vi "String Message add.vi"(4 "Datetime Format":enum16{"Full", "HH:MM:SS"}(ring), 5 "Display":bool=TRUE, 6 "Clear":bool, 7 "String Length":i32=2000, 8 "error in (no error)":errorcluster, 9 "String":string, 10 "Main":string, 11 "Messages":refnum<vi>) -> (0 "error out":errorcluster, 2 "String 2":string, 3 "reference out":refnum<vi>)   [LabVIEW 2021]
doc: "为顶层UI的Message里面累计添加信息。最新的在最上面"
uses:
  <userlib>/sushu/sushu.lvlib
  Z:/UTP_2023/Source_Public/DataBase/DataBase_SQL/DataBase_SQL.lvclass
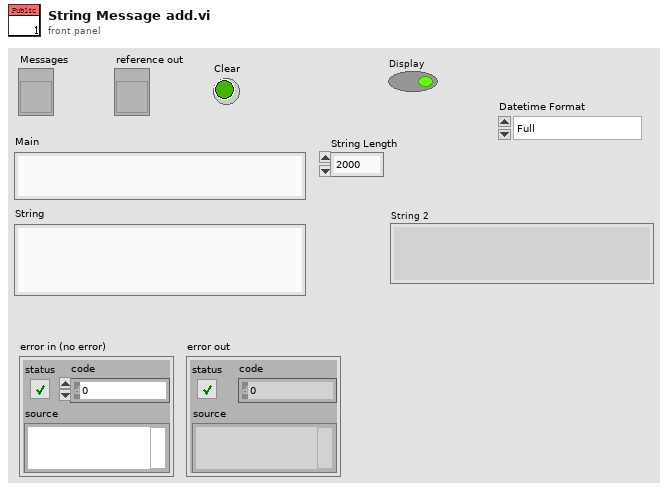
[diagram p1: front panel]
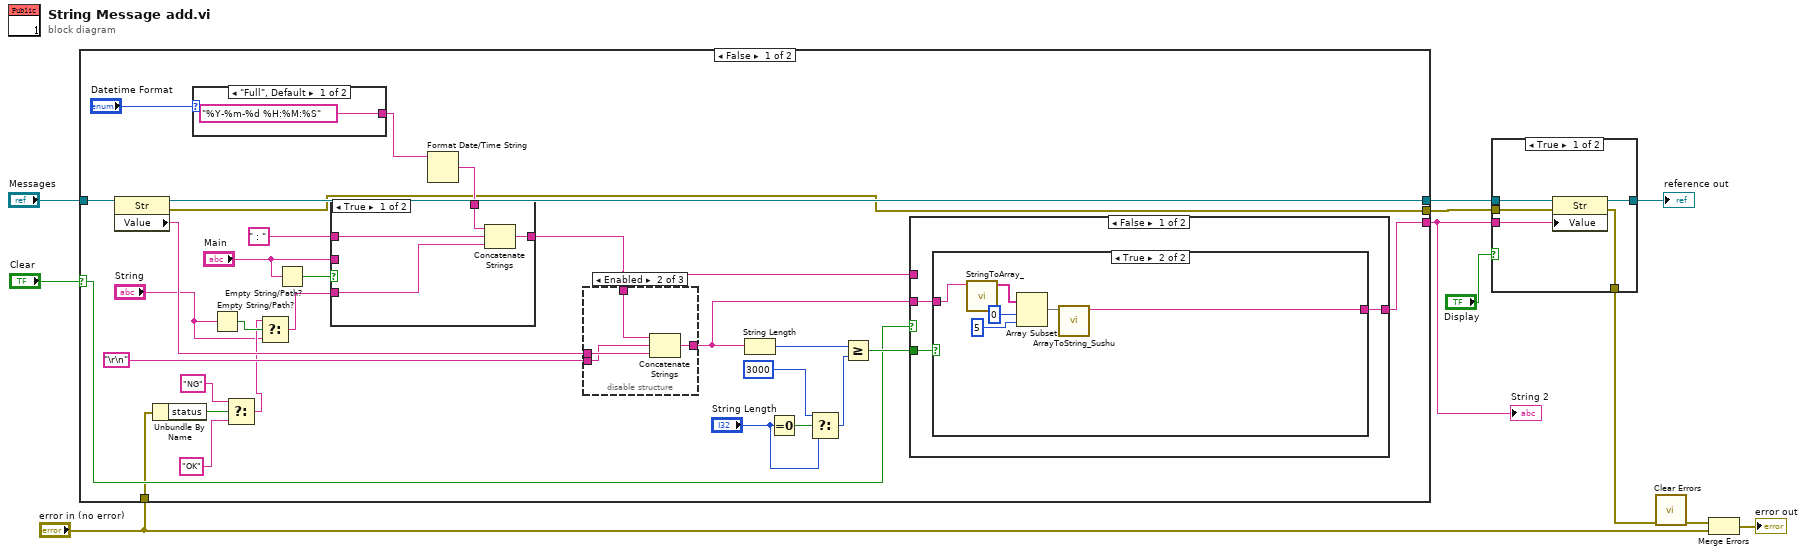
[diagram p0: block diagram]
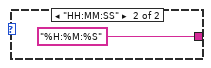
[diagram p3: hidden frame]
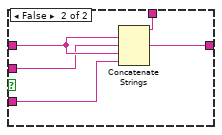
[diagram p6: hidden frame]
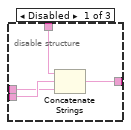
[diagram p7: hidden frame]
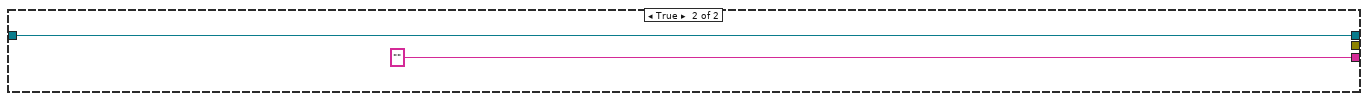
[diagram p9: hidden frame]
diagram:
  n1 = case shown="False" "Clear" {
    selector: "Clear" -> [w24 _]
    tunnel: "Messages" -> [w40 w72]
    tunnel: [w37 w72] -> w10
    tunnel: [w29 "" ("String")] -> w8
    tunnel: "error in (no error)" -> [w22 _]
    tunnel: [w14 _] -> w5
    frame False {
      n2 = property class="Str"(reference=w40) -> (reference out=w37:refnum<vi>, error out=w14:errorcluster, "Value"=w38:string)  [unwired: 1 in]
      n3 = Unbundle By Name(w22) -> ("status"=w21:bool)
      n4 = case shown="\"Full\", Default" "Datetime Format" {
        tunnel: ["%Y-%m-%d %H:%M:%S" ("time format string (%c)") "%H:%M:%S" ("time format string (%c)")] -> w12
        frame "Full", Default {
        }
        frame "HH:MM:SS" {
        }
      }
      n5 = Empty String/Path?(string/path="String") -> (empty?=w18:bool)
      n6 = Select(t="NG" ("string"), s=w21, f="OK" ("string")) -> (s? t:f=w17:string)
      n7 = Select(t=w17, s=w18, f="String") -> (s? t:f=w15:string)
      n8 = Empty String/Path?(string/path="Main") -> (empty?=w26:bool)
      n9 = Format Date/Time String(time format string (%c)=w12) -> (date/time string=w36:string)  [unwired: 2 in]
      n10 = case shown="True" w26 {
        tunnel: [w57 w62] -> w23
        tunnel: w36 -> [w56 w61]
        tunnel: " : " ("string") -> [w55 w60]
        tunnel: w15 -> [w54 w59]
        tunnel: "Main" -> [_ w58]
        frame True {
          n11 = Concatenate Strings(w56, w55, w54) -> (w57:string)
        }
        frame False {
          n12 = Concatenate Strings(w61, w60, w58, w60, w59) -> (w62:string)
        }
      }
      n13 = disable-structure shown="Enabled" {
        disable-tunnel: "\r\n" -> [w66 w68 _]
        disable-tunnel: w38 -> [w65 w70 _]
        disable-tunnel: [w64 w69 _] -> w30
        disable-tunnel: w23 -> [w63 w67 _]
        frame Disabled {
          n14 = Concatenate Strings(w63, w66, w65) -> (w64:string)
        }
        frame Enabled {
          n15 = Concatenate Strings(w67, w68, w70) -> (w69:string)
        }
        frame Disabled {
        }
      }
      n16 = String Length(string=w30) -> (length=w35:i32)
      n17 = Equal To 0?(x="String Length") -> (x = 0?=w34:bool)
      n18 = Select(t=3000 ("y"), s=w34, f="String Length") -> (s? t:f=w31:i32)
      n19 = Greater Or Equal?(x=w35, y=w31) -> (x >= y?=w25:bool)
      n20 = case shown="False" w24 {
        tunnel: w30 -> [w45 _]
        tunnel: [w44 w53] -> w29
        tunnel: w25 -> [w43 _]
        tunnel: w23 -> [_ w53]
        frame False {
          n21 = case shown="True" w43 {
            tunnel: w45 -> [w46 w48]
            tunnel: [w46 w49] -> w44
            frame False {
            }
            frame True {
              n22 = call "StringToArray_.vi"("State Queue"=w48) -> ("Array"=w47:string[])  [unwired: 7 in, 3 out]
              n23 = Array Subset(array=w47, index=0, length=5) -> (w50:string[])
              n24 = call <userlib>:"ArrayToString_Sushu.vi"("Array"=w50) -> ("String"=w49:string)  [unwired: 10 in]
            }
          }
        }
        frame True {
        }
      }
    }
    frame True {
    }
  }
  "String 2" <- w8
  n25 = case shown="True" "Display" {
    tunnel: w10 -> [w77 w79]
    tunnel: [w76 w79] -> w9
    tunnel: w8 -> [w75 _]
    tunnel: w5 -> [w74 w78]
    tunnel: [w73 w78] -> w3
    frame True {
      n26 = property class="Str"(reference=w77, error in=w74, "Value"=w75) -> (reference out=w76:refnum<vi>, error out=w73:errorcluster)
    }
    frame False {
    }
  }
  "reference out" <- w9
  n27 = call <vilib>:"Clear Errors.vi"("error in (no error)"=w3) -> ("error out"=w2:errorcluster)  [unwired: 5 in, 1 out]
  n28 = Merge Errors(w2, "error in (no error)") -> (→"error out":errorcluster)
